vi "Term.vi"(3 "error in":errorcluster, 5 "context in":refnum<class "Context.lvclass">) -> (0 "error out":errorcluster)   [LabVIEW 2025, in "ZeroMQ.lvlib" / "Context.lvclass"]
doc: "Terminates the <b>context</b> fed in. This is a <b>blocking</b> call, and only returns once every socket associated with the context has been terminated.\n\nBecause operations may be pending on sockets, they are given some time (ZMQ_LINGER) to finish before being shut-down by the term call.\n\nThis behaviour can be overwritten by setting <b>reap?</b> to True, which will eliminate all sockets opened by LabVIEW in this context immediately without worrying about close/blocking operations. This may result in unexpected data loss and should only be used in abort situations.\n\nDetailed API documentation: http://api.zeromq.org/3-2:zmq-ctx-destroy"
uses:
  Context.lvclass
  Context.lvclass/Context.ctl
  libzmq-v143-mt-4_3_6/LibZMQ.lvlib
panel:
  # "ØMQ"
  # "labview"
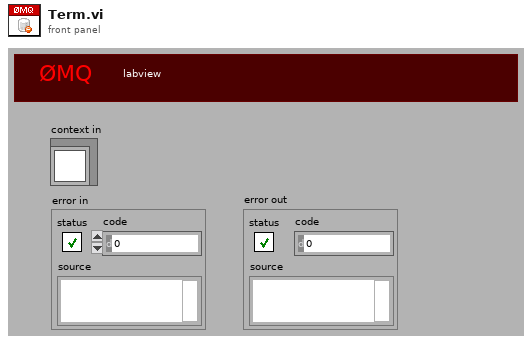
[diagram p1: front panel]
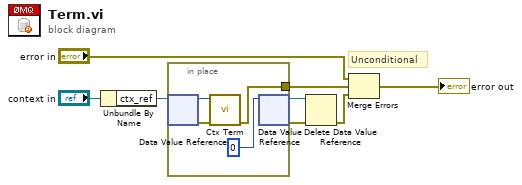
[diagram p0: block diagram]
diagram:
  # "Unconditional"
  n1 = Unbundle By Name("context in") -> ("ctx_ref"=w6:refnum<data-value>)
  n2 = in-place {
    in-place-border: [w9] -> w8
    n3 = in-place-dvr #1(w6) -> (w11:u64, w10:errorcluster)
    n4 = call "Ctx Term.vi"("error in (no error)"=w10, "context_"=w11) -> ("error out"=w9:errorcluster)  [unwired: 9 in]
    n5 = in-place-dvr #1(u64 0 ("data value")) -> (w4:refnum<data-value>, w5:errorcluster)
  }
  n6 = Delete Data Value Reference(data value reference=w4, error in=w5) -> (error out=w1:errorcluster)  [unwired: 1 out]
  n7 = Merge Errors("error in", w8, w1) -> (→"error out":errorcluster)
